vi "Receive Shortcut Menu Selection Event.vi"(8 "error in (no error)":errorcluster, 10 "ShortcutMenuSelectionMsg":refnum<class "ShortcutMenuSelectionMsg.lvclass">, 11 "Test Step Dialog In":refnum<class "Conditional Dialog.lvclass">) -> (0 "error out":errorcluster, 3 "Test Step Dialog Out":refnum<class "Conditional Dialog.lvclass">)   [LabVIEW 2017, in "Conditional Dialog.lvclass"]
doc: "<License>\nCopyright © 2017 Composed Systems, LLC | All rights reserved\nwww.composed.io\n\nAuthor: Ethan Stern <ethan.stern@composed.io>\n\nThis software is provided \"AS IS\" WITHOUT WARRANTIES, either express or implied, AND IS FOR EDUCATIONAL PURPOSES ONLY.\n</License>"
uses:
  Conditional Dialog.lvclass
  <vilib>/gpm_packages/@cs/mva-viewable/Source/ActorEvents/IEventAggregator Messages/ShortcutMenuSelectionMsg/ShortcutMenuSelectionMsg.lvclass
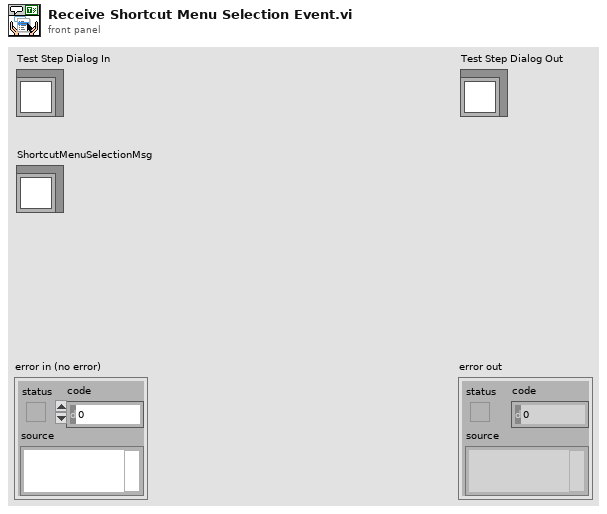
[diagram p1: front panel]
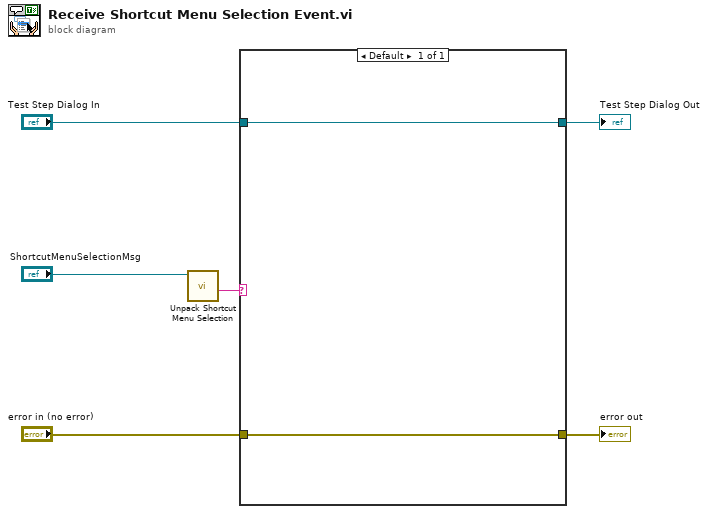
[diagram p0: block diagram]
diagram:
  n1 = call <vilib>:"Unpack Shortcut Menu Selection.vi"("ShortcutMenuSelectionMsg"="ShortcutMenuSelectionMsg") -> ("Item Tag"=w1:string)  [unwired: 3 in, 7 out]
  n2 = case shown="Default" w1 {
    tunnel: [w7] -> w5
    tunnel: "Test Step Dialog In" -> [w7]
    tunnel: [w8] -> w3
    tunnel: "error in (no error)" -> [w8]
    frame Default {
    }
  }
  "error out" <- w3
  "Test Step Dialog Out" <- w5
